vi "subDFD_Get Log Spaced Freq Points.vi"(9 "# points per log freq bin":i32, 10 "end frequency point":dbl, 11 "start frequency point":dbl) -> (3 "freq points":dbl[](array[numeric]))   [LabVIEW 2017]
uses:
  <vilib>/Analysis/1siggen.llb/Ramp Pattern by Samples.vi
  <vilib>/Analysis/NI_AALBase.lvlib
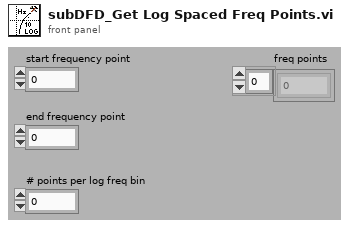
[diagram p1: front panel]
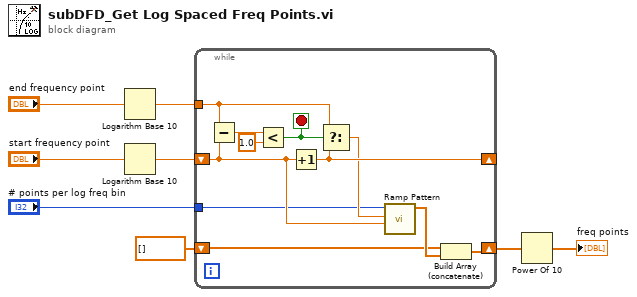
[diagram p0: block diagram]
diagram:
  n1 = Logarithm Base 10(1:"end frequency point") -> (0:w6:dbl)
  n2 = Logarithm Base 10(1:"start frequency point") -> (0:w5:dbl)
  n3 = while {
    tunnel: w6 -> [w17]
    shift-right: [w16] -> _
    shift-left: w5 -> [w14]
    tunnel: "# points per log freq bin" -> [w12]
    shift-right: [w11] -> w2
    shift-left: dbl[] [] -> [w9]
    stop <- w13 stop-if-true
    n4 = Subtract(x=w17, y=w14) -> (x-y=w19:dbl)
    n5 = Less?(x=w19, y=1.0) -> (x < y?=w13:bool)
    n6 = Increment(x=w14) -> (x+1=w16:dbl)
    n7 = Select(t=w17, s=w13, f=w16) -> (s? t:f=w15:dbl)
    n8 = call-poly <vilib>:"Ramp Pattern.vi"("start"=w14, "end"=w15, "samples"=w12) -> ("Ramp Pattern"=w10:dbl[])  [unwired: 7 in, 1 out]
    n9 = Build Array (concatenate)(w9, w10) -> (w11:dbl[])
  }
  n10 = Power Of 10(x=w2) -> (10^x=→"freq points":dbl[])
